vi "Configure Measurement Characteristics (FFT).vi"(0 "VISA resource name":refnum<visa-resource-name>, 5 "Peak Level (-40.0 dB)":dbl=-40.0, 7 "1st Peak Number (1)":i32=1, 9 "2nd Peak Number (1)":i32=1, 11 "error in (no error)":errorcluster) -> (4 "VISA resource name out":refnum<visa-resource-name>, 15 "error out":errorcluster)   [LabVIEW 2020, in "Agilent 90000 Series.lvlib"]
doc: "Sets the peak search threshold value, the first peak number and second peak number for FFT measurements. \n\nThe first peak number and second peak number are used for measurement of FFT delta frequency and FFT delta magnitude."
uses:
  Agilent 90000 Series.lvlib
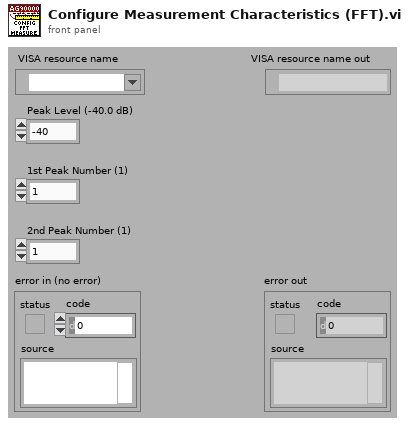
[diagram p1: front panel]
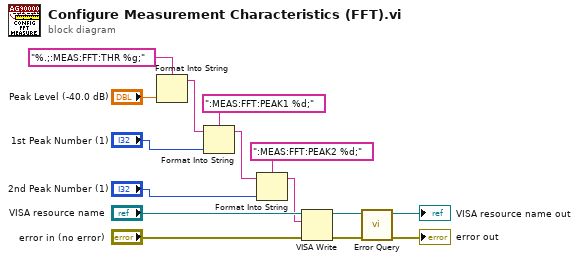
[diagram p0: block diagram]
diagram:
  n1 = Format Into String(format string="%.;:MEAS:FFT:THR %g;", "Peak Level (-40.0 dB)") -> (resulting string=w7:string)  [unwired: 2 in, 1 out]
  n2 = Format Into String(format string=":MEAS:FFT:PEAK1 %d;", initial string=w7, "1st Peak Number (1)") -> (resulting string=w6:string)  [unwired: 1 in, 1 out]
  n3 = Format Into String(format string=":MEAS:FFT:PEAK2 %d;", initial string=w6, "2nd Peak Number (1)") -> (resulting string=w1:string)  [unwired: 1 in, 1 out]
  n4 = VISA Write(VISA resource name="VISA resource name", write buffer=w1, error in (no error)="error in (no error)") -> (VISA resource name out=w11:refnum<visa-resource-name>, error out=w10:errorcluster)  [unwired: 1 out]
  n5 = call "Error Query.vi"("error in (no error)"=w10, "VISA resource name"=w11) -> ("error out"=→"error out":errorcluster, "VISA resource name out"=→"VISA resource name out":refnum<visa-resource-name>)  [unwired: 8 out]
